vi "Encapsulate UDP Message.vi"(5 "source_id":u32, 8 "error in (no error)":errorcluster, 9 "type":string, 10 "Encapsulated Msg":refnum<class "Message.lvclass">, 11 "SequenceCountService":refnum<class "SequenceCountService.lvclass">) -> (0 "error out":errorcluster, 2 "UDP Payload":string)   [LabVIEW 2020, in "Vecto.lvlib"]
uses:
  Vecto.lvlib
  lv-protoc/LV-Proto/Message/Message.lvclass
  SequenceCountService/SequenceCountService.lvclass
  proto/UdpPayload/Data.ctl
  proto/UdpPayload/UdpPayload.lvlib
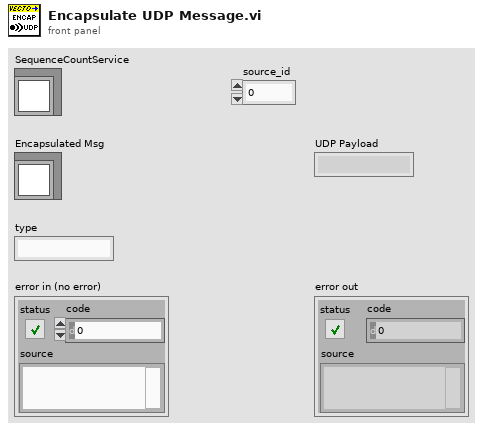
[diagram p1: front panel]
types:
  T1 = typedef "UdpPayload.lvlib/Data.ctl" = cluster{"source_id":u32, "sequence":u32, "timestamp":u64, "type":string, "payload":u8[]}
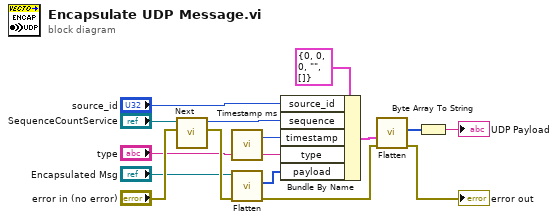
[diagram p0: block diagram]
diagram:
  n1 = call "Next.vi"("error in (no error)"="error in (no error)", "SequenceCountService in"="SequenceCountService") -> ("error out"=w14:errorcluster, "Sequence"=w6:u32)  [unwired: 8 in]
  n2 = call "Timestamp ms.vi"() -> ("Timestamp ms"=w8:u64)  [unwired: 7 in]
  n3 = call-dynamic "Flatten.vi"("error in (no error)"=w14, "Message in"="Encapsulated Msg") -> ("error out"=w2:errorcluster, "Buffer"=w9:u8[])  [unwired: 7 in, 1 out]
  n4 = Bundle By Name(cluster=T1 {"source_id"=0, "sequence"=0, "timestamp"=0, "type"="", "payload"=[]} ("UdpPayload"), "source_id"="source_id", "sequence"=w6, "timestamp"=w8, "type"="type", "payload"=w9) -> (w5:T1)
  n5 = call "Flatten.vi"("error in"=w2, "Data"=w5) -> ("error out"=→"error out":errorcluster, "Buffer"=w4:u8[])  [unwired: 8 in]
  n6 = Byte Array To String(unsigned byte array=w4) -> (string=→"UDP Payload":string)
